vi "getFlags.vi"(11 "PUBREL in":refnum<class "PUBREL.lvclass">) -> (0 "RETAIN":bool, 1 "QoS":T1, 2 "DUP":bool, 3 "PUBREL out":refnum<class "PUBREL.lvclass">)   [LabVIEW 2013, in "PUBREL.lvclass"]
uses:
  PUBREL.lvclass
  QualityOfService -- enum.ctl
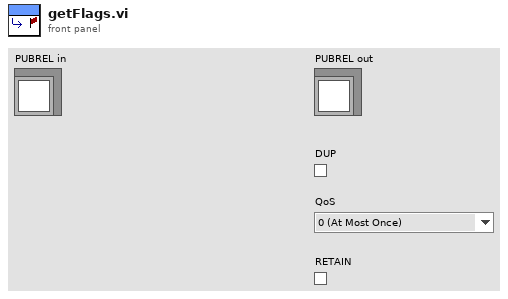
[diagram p1: front panel]
types:
  T1 = typedef "QualityOfService -- enum.ctl" = enum16{"0 (At Most Once)", "1 (At Least Once)", "2 (Exactly Once)"}
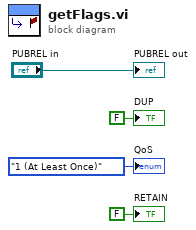
[diagram p0: block diagram]
diagram:
  "PUBREL out" <- "PUBREL in"
  "QoS" <- QualityOfService_--_enum."1 (At Least Once)" ("QoS")
  "DUP" <- FALSE ("DUP")
  "RETAIN" <- FALSE ("RETAIN")
